vi "Set Amp Sweep Stop.vi"(8 "error in (no error)":errorcluster, 10 "Amplitude Sweep Stop (dBm)":dbl, 11 "VISA resource name":refnum<visa-resource-name>) -> (0 "error out":errorcluster, 3 "VISA resource name out":refnum<visa-resource-name>)   [LabVIEW 2012, in "Agilent PSG MXG Series.lvlib"]
uses:
  Agilent PSG MXG Series.lvlib
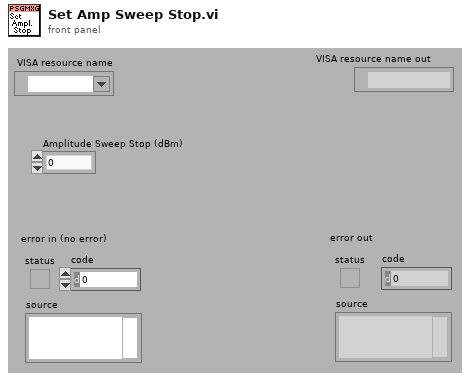
[diagram p1: front panel]
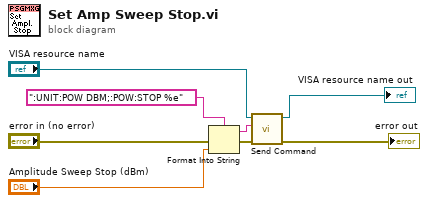
[diagram p0: block diagram]
diagram:
  n1 = Format Into String(format string=":UNIT:POW DBM;:POW:STOP %e", error in="error in (no error)", "Amplitude Sweep Stop (dBm)") -> (resulting string=w2:string, error out=w3:errorcluster)  [unwired: 1 in]
  n2 = call "Send Command.vi"("error in (no error)"=w3, "write buffer"=w2, "VISA resource name"="VISA resource name") -> ("error out"=→"error out":errorcluster, "VISA resource name out"=→"VISA resource name out":refnum<visa-resource-name>)  [unwired: 7 out]
